vi "exercise example 3.vi"() -> ()   [LabVIEW 2021]
panel:
  out "Waveform Chart":dbl(graph)
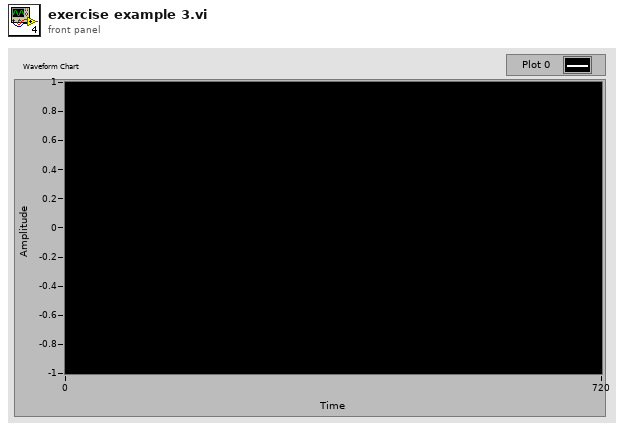
[diagram p1: front panel]
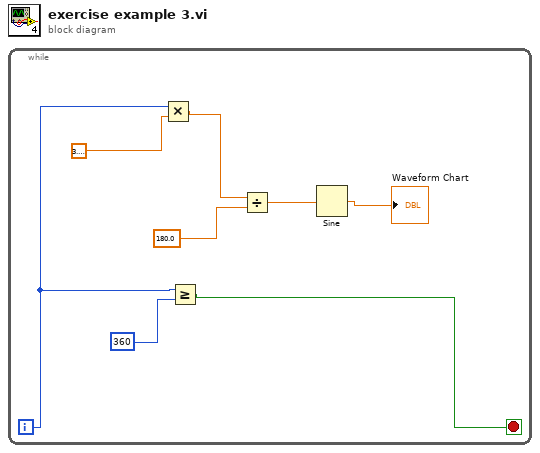
[diagram p0: block diagram]
diagram:
  n1 = while {
    i -> [w8]
    stop <- w4 stop-if-true
    n2 = Multiply(x=w8, y=3.141592653589793) -> (x*y=w6:dbl)
    n3 = Greater Or Equal?(x=w8, y=360) -> (x >= y?=w4:bool)
    n4 = Divide(x=w6, y=180.0) -> (x/y=w5:dbl)
    n5 = Sine(x=w5) -> (sin(x)=→"Waveform Chart":dbl)
  }
